vi "Dashboard Main.vi"() -> ()   [LabVIEW 2013]
uses:
  Dropbox/Robot Code old/2014 Target Detection/TargetType.ctl
  <vilib>/event_ctls.llb/eventvkey.ctl
  <vilib>/Rock Robotics/WPI/Dashboard/WPI_DashboardLogging Global.vi
  <vilib>/Utility/config.llb/Write Key (String).vi
  <vilib>/Utility/config.llb/Write Key (I32).vi
  <vilib>/Utility/config.llb/NI_LVConfig.lvlib
panel:
  in  "Camera Type":enum16{"206", "1011", "1013"}(ring)=enum."1013"
  out "Image Message":string="Timeout in Camera Communications"
  in  "Rec Mode":enum32{"Stop", "Record", "Playback"}(radio)
  in  "Dashboard Tab":T1(tab)
  in  "Camera Settings":T2={"Frame Rate"=30, "Compression"=30, "Size"=1} {"Frame Rate" scale=1.0..30.0; "Size" items=["640x480", "320x240", "160x120"]}
  out "MotorSliders R":cluster{"MotorSlide1":dbl, "MotorSlide2":dbl} {"MotorSlide2" scale=-1.0..1.0 scale format="%#_2e"; "MotorSlide1" scale=-1.0..1.0 scale format="%#_2e"}
  out "MotorChart R":cluster{"Numeric":dbl, "Numeric":dbl}(graph)
  out "MotorSliders L":T3 {"MotorSlide4 2" scale=0.0..14.0 scale format="%#_2e"; "MotorSlide2" scale=-1.0..1.0 scale format="%#_2e"; "MotorSlide1" scale=-1.0..1.0 scale format="%#_2e"}
  out "MotorChart L":T4(graph)
  out "JS1 Z":dbl(slide) scale=-1.0..1.0 scale format="%#_2e"
  out "Joystick 1":cluster{"X":dbl, "Y":dbl}[](graph)
  out "JS Buttons 1":T5
  out "JS2 Z":dbl(slide) scale=-1.0..1.0 scale format="%#_2e"
  out "Joystick 2":cluster{"X":dbl, "Y":dbl}[](graph)
  out "JS Buttons 2":T5
  out "Mode":T6(ring)=enum."Auto Disabled"
  out "Camera IP":string
  in  "DB Camera Config":bool
  out "fps":dbl format="%#.1g"
  out "Mbps":dbl format="%#.1g"
  out "Mbps 2":bool
  out "LED 1":bool
  in  "Score Limit":dbl=70.0
  in  "Slider 1":dbl(slide) scale=0.0..100.0
  out "Goal is hot":bool
  out "Distances":T8(array[cluster])
  in  "Color Components":T9={"Hue"={110.0, 142.0}, "Sat"={138.0, 255.0}, "Val"={139.0, 198.0}} {"Val" scale=0.0..255.0; "Sat" scale=0.0..255.0; "Hue" scale=0.0..255.0 scale format="%#_3g"}
  in  "Checkbox 2":bool
  in  "Checkbox 1":bool
  in  "Test Slider":dbl(slide) scale=0.0..100.0 scale format="%#_3g"
  in  "On/Off":bool caption="Solenoid"
  in  "Test Name":u16(ring) items=["Select the test to run...", "Example Test", "-------------------------------", "List of tests is built in robot code.", "Replace with your own automated tests."]
  in  "Test Tree":string(tree)
  in  "Motor":cluster{"Value":dbl, "Enable":bool} {"Value" scale=-1.0..1.0 scale format="%#_3g"}
  out "Progress":T10 {"Test Progress" scale=0.0..100.0}
  in  "Rev/Fwd":cluster{"Forward":bool, "Reverse":bool}
  in  "Test Ring":u16(ring) items=["Auto", "Fixed indoor", "Fixed outdoor 1", "Fixed outdoor 2", "Fixed fluorescent 1", "Fixed fluorescent 2", "Hold current"]
  in  "Listbox":i32(listbox)
  out "Tree":string(tree)
  out "Camera Image":T11(plugin-control)
  in  "Enable":bool
  # "Left"
  # "Front"
  # "Right"
  # "Battery"
  # "Customize by placing controls and indicators here and name to\nmatch Dashboard Variables on robot."
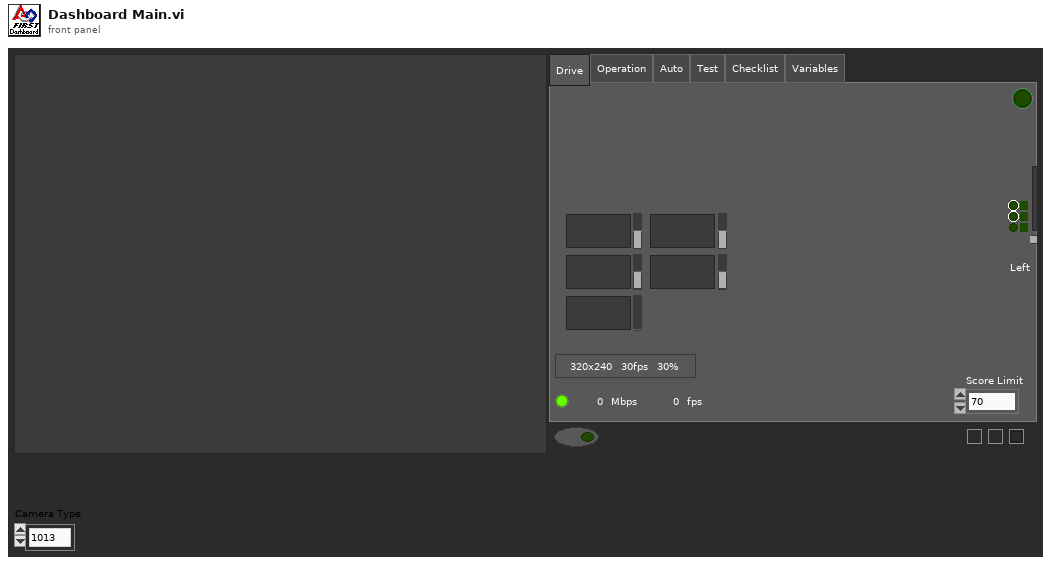
[diagram p1: front panel]
types:
  T1 = enum32{"Drive", "Operation", "Auto", "Test", "Checklist", "Variables"}
  T2 = cluster{"Frame Rate":i32, "Compression":i32, "Size":u16}
  T3 = cluster{"MotorSlide1":dbl, "MotorSlide2":dbl, "MotorSlide4 2":dbl}
  T4 = cluster{"Numeric":dbl, "Numeric":dbl, "Battery":sgl}
  T5 = cluster{bool, bool, bool, bool, bool, bool, bool, bool, bool, bool, bool, bool}
  T6 = enum8{"Tele-Op Disabled", "Tele-Op Enabled", "Auto Disabled", "Auto Enabled", "Test Disabled", "Test Enabled", ""}
  T7 = typedef "TargetType.ctl" = enum16{"Not Hot", "Hot"}
  T8 = cluster{"Distance (ft)":dbl, "Target Center (-1 to 1)":cluster{"X":dbl, "Y":dbl}, "Left":bool, "State":T7}[]
  T9 = cluster{"Hue":cluster{dbl, dbl}, "Sat":cluster{dbl, dbl}, "Val":cluster{dbl, dbl}}
  T10 = cluster{"Test Progress":u8, "Test Progress Text":string}
  T11 = typedef "IMAQ Image.ctl" = refnum<image>
  T12 = typedef "Image Type" = u32
  T13 = cluster{"Digital Inputs":bool[], "Digital Outputs":bool[]}
  T14 = cluster{"Competition mode":bool, "Robot Link":bool, "Autonomous":bool, "Enabled":bool, "E-Stop":bool, "Simulated":bool, "TestMode":bool, "Docked Window":bool}
  T15 = cluster{"Boolean Array[0]":bool, "Boolean Array[1]":bool, "Boolean Array[2]":bool, "Boolean Array[3]":bool, "Boolean Array[4]":bool, "Boolean Array[5]":bool, "Boolean Array[6]":bool, "Boolean Array[7]":bool, "Boolean Array[8]":bool, "Boolean Array[9]":bool, "Boolean Array[10]":bool, "Boolean Array[11]":bool}
  T16 = cluster{"Horizontal":bool, "Aspect Score":dbl, "Rect Score":dbl, cluster{"Left":dbl, "Top":dbl, "Right":dbl, "Bottom":dbl}, "Equiv H":dbl, "Equiv V":dbl}[]
  T17 = cluster{"Scores":cluster{"Total":dbl, "Left":dbl, "Right":dbl, "Ratio":dbl, "Vertical":dbl, "index":i32, "State":T7}, "Verticals":cluster{"Horizontal?":bool, "Aspect Score":dbl, "Rect Score":dbl, cluster{"Left":dbl, "Top":dbl, "Right":dbl, "Bottom":dbl}, "Equiv H":dbl, "Equiv V":dbl}, "Horizontals":cluster{"Horizontal?":bool, "Aspect Score":dbl, "Rect Score":dbl, cluster{"Left":dbl, "Top":dbl, "Right":dbl, "Bottom":dbl}, "Equiv H":dbl, "Equiv V":dbl}, "Validated":bool}[]
  T18 = cluster{"Scores":cluster{"Total":dbl, "Left":dbl, "Right":dbl, "Ratio":dbl, "Vertical":dbl, "index":i32, "State":T7}, "Verticals":cluster{"Horizontal?":bool, "Aspect Score":dbl, "Rect Score":dbl, cluster{"Left":dbl, "Top":dbl, "Right":dbl, "Bottom":dbl}, "Equiv H":dbl, "Equiv V":dbl}, "Horizontals":cluster{"Horizontal?":bool, "Aspect Score":dbl, "Rect Score":dbl, cluster{"Left":dbl, "Top":dbl, "Right":dbl, "Bottom":dbl}, "Equiv H":dbl, "Equiv V":dbl}, "Distance (ft)":dbl, "Target Center (-1 to 1)":cluster{"X":dbl, "Y":dbl}}[]
  T19 = cluster{"Target Info[0]":cluster{"Scores":cluster{"Total":dbl, "Left":dbl, "Right":dbl, "Ratio":dbl, "Vertical":dbl, "index":i32, "State":T7}, "Verticals":cluster{"Horizontal?":bool, "Aspect Score":dbl, "Rect Score":dbl, cluster{"Left":dbl, "Top":dbl, "Right":dbl, "Bottom":dbl}, "Equiv H":dbl, "Equiv V":dbl}, "Horizontals":cluster{"Horizontal?":bool, "Aspect Score":dbl, "Rect Score":dbl, cluster{"Left":dbl, "Top":dbl, "Right":dbl, "Bottom":dbl}, "Equiv H":dbl, "Equiv V":dbl}, "Distance (ft)":dbl, "Target Center (-1 to 1)":cluster{"X":dbl, "Y":dbl}}, "Target Info[1]":cluster{"Scores":cluster{"Total":dbl, "Left":dbl, "Right":dbl, "Ratio":dbl, "Vertical":dbl, "index":i32, "State":T7}, "Verticals":cluster{"Horizontal?":bool, "Aspect Score":dbl, "Rect Score":dbl, cluster{"Left":dbl, "Top":dbl, "Right":dbl, "Bottom":dbl}, "Equiv H":dbl, "Equiv V":dbl}, "Horizontals":cluster{"Horizontal?":bool, "Aspect Score":dbl, "Rect Score":dbl, cluster{"Left":dbl, "Top":dbl, "Right":dbl, "Bottom":dbl}, "Equiv H":dbl, "Equiv V":dbl}, "Distance (ft)":dbl, "Target Center (-1 to 1)":cluster{"X":dbl, "Y":dbl}}, "Target Info[2]":cluster{"Scores":cluster{"Total":dbl, "Left":dbl, "Right":dbl, "Ratio":dbl, "Vertical":dbl, "index":i32, "State":T7}, "Verticals":cluster{"Horizontal?":bool, "Aspect Score":dbl, "Rect Score":dbl, cluster{"Left":dbl, "Top":dbl, "Right":dbl, "Bottom":dbl}, "Equiv H":dbl, "Equiv V":dbl}, "Horizontals":cluster{"Horizontal?":bool, "Aspect Score":dbl, "Rect Score":dbl, cluster{"Left":dbl, "Top":dbl, "Right":dbl, "Bottom":dbl}, "Equiv H":dbl, "Equiv V":dbl}, "Distance (ft)":dbl, "Target Center (-1 to 1)":cluster{"X":dbl, "Y":dbl}}, "Target Info[3]":cluster{"Scores":cluster{"Total":dbl, "Left":dbl, "Right":dbl, "Ratio":dbl, "Vertical":dbl, "index":i32, "State":T7}, "Verticals":cluster{"Horizontal?":bool, "Aspect Score":dbl, "Rect Score":dbl, cluster{"Left":dbl, "Top":dbl, "Right":dbl, "Bottom":dbl}, "Equiv H":dbl, "Equiv V":dbl}, "Horizontals":cluster{"Horizontal?":bool, "Aspect Score":dbl, "Rect Score":dbl, cluster{"Left":dbl, "Top":dbl, "Right":dbl, "Bottom":dbl}, "Equiv H":dbl, "Equiv V":dbl}, "Distance (ft)":dbl, "Target Center (-1 to 1)":cluster{"X":dbl, "Y":dbl}}, "Target Info[4]":cluster{"Scores":cluster{"Total":dbl, "Left":dbl, "Right":dbl, "Ratio":dbl, "Vertical":dbl, "index":i32, "State":T7}, "Verticals":cluster{"Horizontal?":bool, "Aspect Score":dbl, "Rect Score":dbl, cluster{"Left":dbl, "Top":dbl, "Right":dbl, "Bottom":dbl}, "Equiv H":dbl, "Equiv V":dbl}, "Horizontals":cluster{"Horizontal?":bool, "Aspect Score":dbl, "Rect Score":dbl, cluster{"Left":dbl, "Top":dbl, "Right":dbl, "Bottom":dbl}, "Equiv H":dbl, "Equiv V":dbl}, "Distance (ft)":dbl, "Target Center (-1 to 1)":cluster{"X":dbl, "Y":dbl}}, "Target Info[5]":cluster{"Scores":cluster{"Total":dbl, "Left":dbl, "Right":dbl, "Ratio":dbl, "Vertical":dbl, "index":i32, "State":T7}, "Verticals":cluster{"Horizontal?":bool, "Aspect Score":dbl, "Rect Score":dbl, cluster{"Left":dbl, "Top":dbl, "Right":dbl, "Bottom":dbl}, "Equiv H":dbl, "Equiv V":dbl}, "Horizontals":cluster{"Horizontal?":bool, "Aspect Score":dbl, "Rect Score":dbl, cluster{"Left":dbl, "Top":dbl, "Right":dbl, "Bottom":dbl}, "Equiv H":dbl, "Equiv V":dbl}, "Distance (ft)":dbl, "Target Center (-1 to 1)":cluster{"X":dbl, "Y":dbl}}, "Target Info[6]":cluster{"Scores":cluster{"Total":dbl, "Left":dbl, "Right":dbl, "Ratio":dbl, "Vertical":dbl, "index":i32, "State":T7}, "Verticals":cluster{"Horizontal?":bool, "Aspect Score":dbl, "Rect Score":dbl, cluster{"Left":dbl, "Top":dbl, "Right":dbl, "Bottom":dbl}, "Equiv H":dbl, "Equiv V":dbl}, "Horizontals":cluster{"Horizontal?":bool, "Aspect Score":dbl, "Rect Score":dbl, cluster{"Left":dbl, "Top":dbl, "Right":dbl, "Bottom":dbl}, "Equiv H":dbl, "Equiv V":dbl}, "Distance (ft)":dbl, "Target Center (-1 to 1)":cluster{"X":dbl, "Y":dbl}}, "Target Info[7]":cluster{"Scores":cluster{"Total":dbl, "Left":dbl, "Right":dbl, "Ratio":dbl, "Vertical":dbl, "index":i32, "State":T7}, "Verticals":cluster{"Horizontal?":bool, "Aspect Score":dbl, "Rect Score":dbl, cluster{"Left":dbl, "Top":dbl, "Right":dbl, "Bottom":dbl}, "Equiv H":dbl, "Equiv V":dbl}, "Horizontals":cluster{"Horizontal?":bool, "Aspect Score":dbl, "Rect Score":dbl, cluster{"Left":dbl, "Top":dbl, "Right":dbl, "Bottom":dbl}, "Equiv H":dbl, "Equiv V":dbl}, "Distance (ft)":dbl, "Target Center (-1 to 1)":cluster{"X":dbl, "Y":dbl}}, "Target Info[8]":cluster{"Scores":cluster{"Total":dbl, "Left":dbl, "Right":dbl, "Ratio":dbl, "Vertical":dbl, "index":i32, "State":T7}, "Verticals":cluster{"Horizontal?":bool, "Aspect Score":dbl, "Rect Score":dbl, cluster{"Left":dbl, "Top":dbl, "Right":dbl, "Bottom":dbl}, "Equiv H":dbl, "Equiv V":dbl}, "Horizontals":cluster{"Horizontal?":bool, "Aspect Score":dbl, "Rect Score":dbl, cluster{"Left":dbl, "Top":dbl, "Right":dbl, "Bottom":dbl}, "Equiv H":dbl, "Equiv V":dbl}, "Distance (ft)":dbl, "Target Center (-1 to 1)":cluster{"X":dbl, "Y":dbl}}}
  T20 = cluster{cluster{dbl, dbl}, cluster{dbl, dbl}, cluster{dbl, dbl}}
  T21 = typedef "NI_LVConfig.lvlib/Config Data RefNum.ctl" = refnum<k1>
  T22 = typedef "eventvkey.ctl" = enum16{"ASCII", "Enter", "Return", "Shift", "Ctrl", "Alt", "Cmd", "Opt", "Caps", "NumLock", "Clear", "Break", "Up", "Down", "Left", "Right", "Insert", "Delete", "Home", "End", "PageUp", "PageDown", "Escape", "Help", "Pause", "ScrollLock", "F1", "F2", "F3", "F4", "F5", "F6", "F7", "F8", "F9", "F10", "F11", "F12", "F13", "F14", "F15", "F16", "F17", "F18", "F19", "F20", "F21", "F22", "F23", "F24", "Play", "VolumeUp", "VolumeDown", "Mute", "Two Byte Char"}
  T23 = cluster{"Image Size":bool, "Image Type":bool, "Pixel Value":bool, "ROI Information":bool, "Zoom Factor":bool}
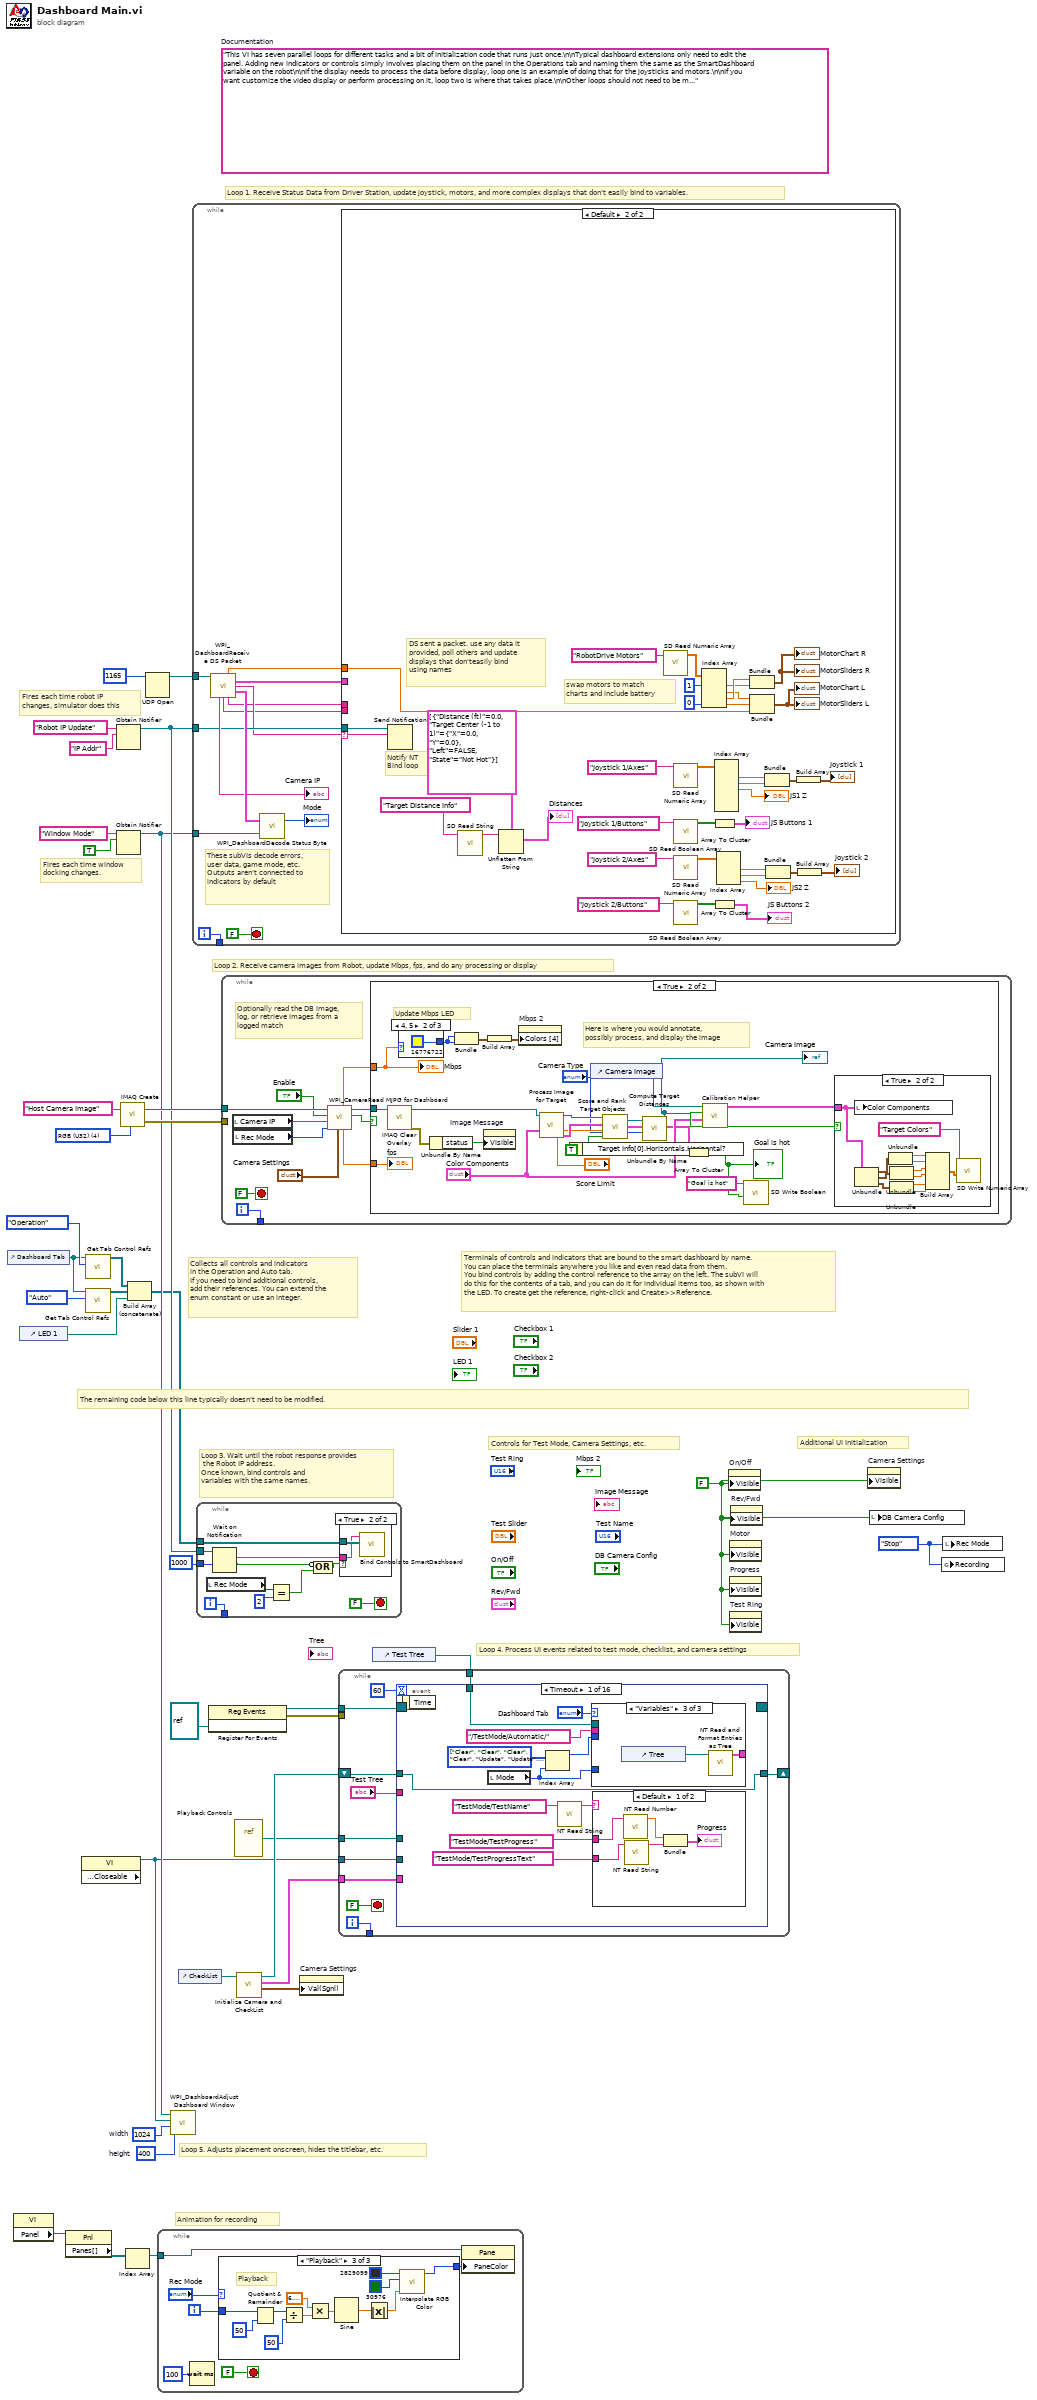
[diagram p0: block diagram]
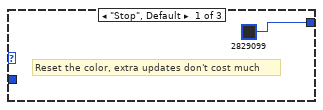
[diagram p2: hidden frame]
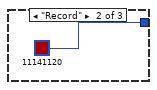
[diagram p3: hidden frame]
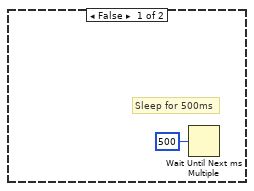
[diagram p5: hidden frame]
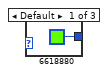
[diagram p7: hidden frame]
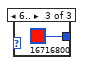
[diagram p8: hidden frame]
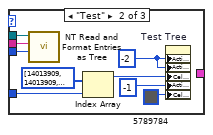
[diagram p10: hidden frame]
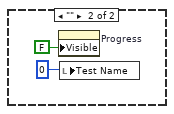
[diagram p11: hidden frame]
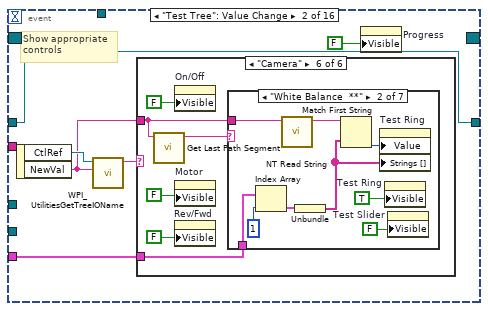
[diagram p12: hidden frame]
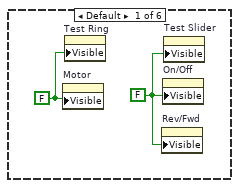
[diagram p13: hidden frame]
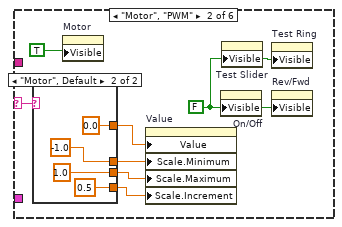
[diagram p14: hidden frame]
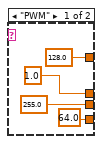
[diagram p15: hidden frame]
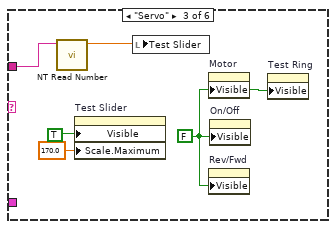
[diagram p16: hidden frame]
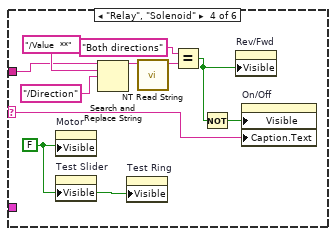
[diagram p17: hidden frame]
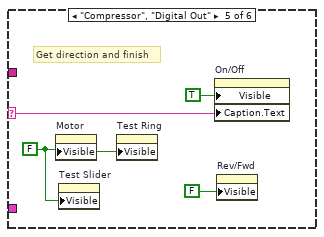
[diagram p18: hidden frame]
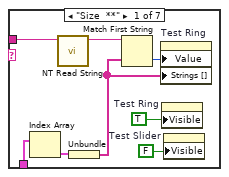
[diagram p19: hidden frame]
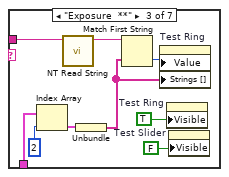
[diagram p20: hidden frame]
diagram:
  w8 = enum32{"Stop", "Record", "Playback"}."Stop" ("Rec Mode")
  w11 = 400  # height
  w12 = 1024  # width
  w25 = FALSE ("Visible")
  (unwired) "This VI has seven parallel loops for different tasks and a bit of initialization code that runs just once.\n\nTypical dashboard extensions only need to edit the panel. Adding new indicators or controls simply involves placing them on the panel in the Operations tab and naming them the same as the SmartDashboard variable on the robot\n\nIf the display needs to process the data before display, loop one is an example of doing that for the joysticks and motors.\n\nIf you want customize the video display or perform processing on it, loop two is where that takes place.\n\nOther loops should not need to be modified. They are pretty standard, and document the task they perform."  # Documentation
  w35 = T12 4 items=["Grayscale (U8)", "Grayscale (I16)", "Grayscale (SGL)", "Complex (CSG)", "RGB (U32)", "HSL (U32)", "RGB (U64)"] ("Image Type")
  # "Controls for Test Mode, Camera Settings, etc."
  # "Additional UI Initialization"
  # "Animation for recording"
  # "Fires each time robot IP\nchanges, simulator does this"
  # "Fires each time window\ndocking changes."
  # "Collects all controls and indicators\nin the Operation and Auto tab.\nIf you need to bind additional controls,\nadd their references. You can extend the\nenum constant or use an integer."
  # "The remaining code below this line typically doesn't need to be modified."
  # "Loop 4. Process UI events related to test mode, checklist, and camera settings"
  # "Terminals of controls and indicators that are bound to the smart dashboard by name.\nYou can place the terminals anywhere you like and even read data from them.\nYou bind controls by adding the control reference to the array on the left. The subVI will\ndo this for the contents of a tab, and you can do it for individual items too, as shown with\nthe LED. To create get the reference, right-click and Create>>Reference."
  # "Loop 3. Wait until the robot response provides\n the Robot IP address.\nOnce known, bind controls and\nvariables with the same names."
  # "Loop 5. Adjusts placement onscreen, hides the titlebar, etc."
  # "Loop 1. Receive Status Data from Driver Station, update joystick, motors, and more complex displays that don't easily bind to variables."
  # "Loop 2. Receive camera images from Robot, update Mbps, fps, and do any processing or display"
  n1 = control-ref of="Dashboard Tab"() -> (w6:refnum<vi>)
  n2 = property class="VI"() -> ("Panel"=w19:refnum<vi>)  [unwired: 2 in, 2 out]
  n3 = control-ref of="LED 1"() -> (w1:refnum<vi>)
  n4 = property class="Pnl"(reference=w19) -> ("Panes[]"=w20:refnum<vi>[])  [unwired: 1 in, 2 out]
  n5 = property class="VI" props=["Front Panel.Closeable"]() -> (reference out=w7:refnum<vi>)  [unwired: 2 in, 2 out]
  n6 = call <vilib>:"Get Tab Control Refs.vi"("Page Index"=T1."Operation" ("Dashboard Tab"), "TabControl in"=w6) -> ("ControlsOnPage"=w4:refnum<vi>[])  [unwired: 9 in]
  n7 = call <vilib>:"Get Tab Control Refs.vi"("Page Index"=T1."Auto" ("Dashboard Tab"), "TabControl in"=w6) -> ("ControlsOnPage"=w5:refnum<vi>[])  [unwired: 9 in]
  n8 = Obtain Notifier(name (unnamed)="Robot IP Update", notification data type="IP Addr" ("name (unnamed)")) -> (notifier out=w29:refnum<notifier>)  [unwired: 2 in, 2 out]
  n9 = Obtain Notifier(name (unnamed)="Window Mode", notification data type=TRUE) -> (notifier out=w10:refnum<notifier>)  [unwired: 2 in, 2 out]
  n10 = call "IMAQ Create"("Image Name"="Host Camera Image", "Image Type"=w35) -> ("New Image"=w33:T11, "error out"=w32:errorcluster)  [unwired: 2 in, 1 out]
  n11 = Index Array(array=w20) -> (element=w18:refnum<vi>)  [unwired: 1 in]
  n12 = Build Array (concatenate)(w4, w5, w1) -> (w3:refnum<vi>[])
  n13 = UDP Open(11:u16 1165 ("port")) -> (port=w36:refnum<k16>)  [unwired: 2 in, 4 out]
  n14 = while {
    tunnel: w18 -> [w39]
    i -> [w42]
    stop <- FALSE stop-if-true
    n15 = Wait (ms)(milliseconds to wait=u32 100) -> ()  [unwired: 1 out]
    n16 = case shown="\"Playback\"" "Rec Mode" {
      tunnel: w42 -> [_ _ w57]
      tunnel: [u32 2829099 ("Base Color") u32 11141120 ("Target Color") w46] -> w38
      frame "Stop", Default {
        # "Reset the color, extra updates don't cost much"
      }
      frame "Record" {
      }
      frame "Playback" {
        # "Playback"
        n17 = Quotient & Remainder(x=w57, y=u32 50 ("milliseconds to wait")) -> (x-y*floor(x/y)=w53:u32)  [unwired: 1 out]
        n18 = Divide(x=w53, y=u32 50 ("milliseconds to wait")) -> (x/y=w50:dbl)
        n19 = Multiply(x=6.283185307179586, y=w50) -> (x*y=w55:dbl)
        n20 = Sine(x=w55) -> (sin(x)=w54:dbl)
        n21 = Absolute Value(x=w54) -> (abs(x)=w47:dbl)
        n22 = call "Interpolate RGB Color.vi"("Proportion"=w47, "Target Color"=u32 30976, "Base Color"=u32 2829099) -> ("Result Color"=w46:u32)  [unwired: 8 in]
      }
    }
    n23 = property class="Pane"(reference=w39, "PaneColor"=w38) -> ()  [unwired: 1 in, 2 out]
  }
  n24 = call <vilib>:"WPI_DashboardAdjust Dashboard Window.vi"("height"=w11, "width"=w12, "reference in"=w7, "Notifier in"=w10) -> ()  [unwired: 8 in]
  n25 = control-ref of="CheckList"() -> (w9:refnum<vi>)
  n26 = while {
    tunnel: w36 -> [w68]
    tunnel: w29 -> [w63]
    tunnel: w10 -> [w67]
    tunnel: [w64] -> _
    i -> [w64]
    stop <- FALSE stop-if-true
    # "These subVIs decode errors, user data, game mode, etc.\nOutputs aren't connected to indicators by default"
    n27 = call <vilib>:"WPI_DashboardReceive DS Packet.vi"("Recv Socket"=w68) -> ("Battery"=w58:sgl, "Driver Station"=w59:T13, "Robot IP Address"=w62:string, "Status"=w69:T14, "Camera IP Address"=→"Camera IP":string, "Low Priority User Data"=w61:string, "High Priority User Data"=w60:string)  [unwired: 1 in, 7 out]
    n28 = call <vilib>:"WPI_DashboardDecode Status Byte.vi"("Window Mode Notifier"=w67, "Status"=w69) -> ("Mode"=→"Mode":T6)  [unwired: 1 out]
    n29 = case shown="Default" w62 {
      selector: w62 -> [_ w85]
      tunnel: w63 -> [_ w86]
      tunnel: w61 -> [_ _]
      tunnel: w60 -> [_ _]
      tunnel: w59 -> [_ _]
      tunnel: w58 -> [_ w84]
      frame "0.0.0.0" {
        # "DS not sending packets, or no robot exists yet.\nDon't poll the variables"
      }
      frame Default {
        # "Notify NT\nBind loop"
        # "DS sent a packet. use any data it\nprovided, poll others and update\ndisplays that don'teasily bind\nusing names"
        # "swap motors to match\ncharts and include battery"
        n30 = Send Notification(notification=w85, notifier=w86) -> ()  [unwired: 1 in, 2 out]
        n31 = call <vilib>:"SD Read String.vi"("Name"="Target Distance Info") -> ("String"=w74:string)  [unwired: 8 in, 2 out]
        n32 = Unflatten From String(type=T8 [{"Distance (ft)"=0.0, "Target Center (-1 to 1)"={"X"=0.0, "Y"=0.0}, "Left"=FALSE, "State"=enum."Not Hot"}] ("Distances"), binary string=w74) -> (value=→"Distances":T8)  [unwired: 3 in, 2 out]
        n33 = call <vilib>:"SD Read Numeric Array.vi"("Name"="RobotDrive Motors") -> ("Numeric Array"=w83:dbl[])  [unwired: 8 in, 2 out]
        n34 = call <vilib>:"SD Read Numeric Array.vi"("Name"="Joystick 1/Axes") -> ("Numeric Array"=w102:dbl[])  [unwired: 8 in, 2 out]
        n35 = call <vilib>:"SD Read Boolean Array.vi"("Name"="Joystick 1/Buttons") -> ("Boolean Array"=w104:bool[])  [unwired: 8 in, 2 out]
        n36 = call <vilib>:"SD Read Numeric Array.vi"("Name"="Joystick 2/Axes") -> ("Numeric Array"=w96:dbl[])  [unwired: 8 in, 2 out]
        n37 = call <vilib>:"SD Read Boolean Array.vi"("Name"="Joystick 2/Buttons") -> ("Boolean Array"=w95:bool[])  [unwired: 8 in, 2 out]
        n38 = Index Array(array=w83, index #1=1, index #4=0) -> (element #1=w79:dbl, element #2=w78:dbl, element #3=w80:dbl, element #4=w75:dbl)  [unwired: 2 in]
        n39 = Array To Cluster(array=w104) -> (cluster=→"JS Buttons 1":T15)
        n40 = Array To Cluster(array=w95) -> (cluster=→"JS Buttons 2":T15)
        n41 = Index Array(array=w102) -> (element #1=w99:dbl, element #2=w100:dbl, element #3=→"JS1 Z":dbl)  [unwired: 6 in, 3 out]
        n42 = Index Array(array=w96) -> (element #1=w91:dbl, element #2=w90:dbl, element #3=→"JS2 Z":dbl)  [unwired: 3 in]
        n43 = Bundle("Numeric"=w80, "Numeric"=w79) -> (→"MotorChart R" →"MotorSliders R":cluster{"Numeric":dbl, "Numeric":dbl})  [unwired: 1 in]
        n44 = Bundle("Numeric"=w78, "Numeric"=w75, "Battery"=w84) -> (→"MotorChart L" →"MotorSliders L":T4)  [unwired: 1 in]
        n45 = Bundle("Numeric"=w99, "Numeric"=w100) -> (w98:cluster{"Numeric":dbl, "Numeric":dbl})  [unwired: 1 in]
        n46 = Bundle("Numeric"=w91, "Numeric"=w90) -> (w92:cluster{"Numeric":dbl, "Numeric":dbl})  [unwired: 1 in]
        n47 = Build Array(w98) -> (→"Joystick 1":cluster{"Numeric":dbl, "Numeric":dbl}[])
        n48 = Build Array(w92) -> (→"Joystick 2":cluster{"Numeric":dbl, "Numeric":dbl}[])
      }
    }
  }
  n49 = while {
    tunnel: w3 -> [w118]
    tunnel: w29 -> [w116]
    tunnel: [w114] -> _
    tunnel: u32 1000 ("milliseconds to wait") -> [w113]
    i -> [w114]
    stop <- FALSE stop-if-true
    n50 = local read "Rec Mode"() -> (w109:enum32{"Stop", "Record", "Playback"})
    n51 = Wait on Notification(notifier=w116, timeout in ms (-1)=w113) -> (notification=w115:string, timed out?=w111:bool)  [unwired: 2 in, 2 out]
    n52 = Equal?(x=w109, y=u16 2 ("Rec Mode")) -> (x = y?=w110:bool)
    n53 = Compound Arithmetic op=OR(invert w111, w110) -> (w112:bool)
    n54 = case shown="True" w112 {
      tunnel: w118 -> [_ w120]
      tunnel: w115 -> [_ w119]
      frame False {
      }
      frame True {
        n55 = call <vilib>:"Bind Controls to SmartDashboard.vi"("Bound Control Refs"=w120, "Server IP Address"=w119) -> ()  [unwired: 10 in]
      }
    }
  }
  n56 = register-events(refnum<vi> refnum) -> (reference out=w16:refnum<event-registration>, error out=w15:errorcluster)  [unwired: 2 in]
  n57 = while {
    tunnel: w33 -> [w129]
    tunnel: w32 -> [_]
    tunnel: [w130] -> _
    i -> [w130]
    stop <- FALSE stop-if-true
    # "Optionally read the DB image,\nlog, or retrieve images from a\nlogged match"
    n58 = local read "Camera IP"() -> (w122:string)
    n59 = local read "Rec Mode"() -> (w121:enum32{"Stop", "Record", "Playback"})
    n60 = call <vilib>:"WPI_CameraRead MJPG for Dashboard.vi"("Camera Settings"="Camera Settings", "Rec Mode"=w121, "Camera IP"=w122, "Enable"="Enable", "Refnum in"=w129) -> ("Active"=w126:bool, "Refnum out"=w128:T11, "FPS"=w125:dbl, "Bandwidth (Mbps)"=w124:dbl)  [unwired: 3 in]
    n61 = case shown="True" w126 {
      tunnel: w128 -> [_ w152]
      tunnel: w124 -> [_ w151]
      tunnel: w125 -> [_ w150]
      frame False {
        # "Sleep for 500ms"
        n62 = Wait Until Next ms Multiple(millisecond multiple=u32 500) -> ()  [unwired: 1 out]
      }
      frame True {
        # "Here is where you would annotate,\npossibly process, and display the image"
        # "Update Mbps LED"
        n63 = call "IMAQ Clear Overlay"("Image"=w152) -> ("error out"=w156:errorcluster, "Image Out"=w145:T11)  [unwired: 2 in, 7 out]
        n64 = case shown="4, 5" w151 {
          tunnel: [u32 6618880 ("Color Box") u32 16776722 ("Color Box") u32 16716800 ("Color Box")] -> w153
          frame Default {
          }
          frame 4, 5 {
          }
          frame 6.. {
          }
        }
        n65 = Unbundle By Name(w156) -> ("status"=w157:bool)
        n66 = Bundle("Color Box"=w153, "Color Box"=w153) -> (w155:cluster{"Color Box":u32, "Color Box":u32})  [unwired: 1 out]
        n67 = property on="Image Message" class="Str"("Visible"=w157) -> ()  [unwired: 2 in, 2 out]
        n68 = Build Array(w155) -> (w154:cluster{"Color Box":u32, "Color Box":u32}[])
        n69 = property on="Mbps 2" class="Bool (strict)"("Colors [4]"=w154) -> ()  [unwired: 2 in, 2 out]
        n70 = call "Process Image for Target.vi"("Src Image"=w145, "Color Components"="Color Components") -> ("Src Image Out"=w144:T11, "Particles"=w143:T16)  [unwired: 11 in, 1 out]
        n71 = control-ref of="Camera Image"() -> (w149:refnum<vi>)
        n72 = call "Score and Rank Target Objects.vi"("Annotate"=TRUE, "Score Limit"="Score Limit", "Particles"=w143, "Image in"=w144) -> ("Target Info"=w142:T17, "Annotated Image"=w141:T11)  [unwired: 6 in]
        n73 = call "Compute Target Distances.vi"("Camera Type"="Camera Type", "Target Info"=w142, "Image in"=w141) -> ("Target Info"=w136:T18, "Image out"=w140:T11)  [unwired: 6 in, 1 out]
        "Camera Image" <- w140
        n74 = Array To Cluster(array=w136) -> (cluster=w135:T19)
        n75 = Unbundle By Name(w135) -> ("Target Info[0].Horizontals.Horizontal?"=w134:bool)
        "Goal is hot" <- w134
        n76 = call "Calibration Helper.vi"("Color Components"="Color Components", "Image"=w140, "Image Ctl Refnum"=w149) -> ("Changed"=w147:bool, "output color"=w148:T20)  [unwired: 7 in]
        n77 = call <vilib>:"SD Write Boolean.vi"("Boolean"=w134, "Name"="Goal is hot") -> ()  [unwired: 8 in, 2 out]
        n78 = case shown="True" w147 {
          tunnel: w148 -> [_ w169]
          frame False {
          }
          frame True {
            n79 = local write "Color Components"(w169) -> ()
            n80 = Unbundle(w169) -> (w168:cluster{dbl, dbl}, w167:cluster{dbl, dbl}, w166:cluster{dbl, dbl})
            n81 = Unbundle(w168) -> (w165:dbl, w164:dbl)
            n82 = Unbundle(w167) -> (w163:dbl, w162:dbl)
            n83 = Unbundle(w166) -> (w161:dbl, w160:dbl)
            n84 = Build Array(w165, w164, w163, w162, w161, w160) -> (w159:dbl[])
            n85 = call <vilib>:"SD Write Numeric Array.vi"("Numeric Array"=w159, "Name"="Target Colors") -> ()  [unwired: 8 in, 2 out]
          }
        }
        "Mbps" <- w151
        "fps" <- w150
      }
    }
  }
  n86 = vi-ref "Playback Controls.vi"() -> (w17:refnum<vi>)
  n87 = call "Initialize Camera and CheckList.vi"("ListBox in"=w9) -> ("Cluster"=w23:cluster{"value":i32, "value":i32, "index":i32}, "Array"=w24:cluster{string[]}[], "File Refnum"=w22:T21)  [unwired: 8 in]
  n88 = property on="Camera Settings" class="Clust (strict)"("Val(Sgnl)"=w23) -> ()  [unwired: 2 in, 2 out]
  n89 = control-ref of="Test Tree"() -> (w21:refnum<vi>)
  n90 = while {
    tunnel: w24 -> [w180]
    shift-right: [w179] -> _
    shift-left: w22 -> [w178]
    tunnel: [w177] -> _
    tunnel: w21 -> [w176]
    tunnel: w17 -> [w175]
    tunnel: w16 -> [w174]
    tunnel: w15 -> [_]
    tunnel: w7 -> [w173]
    i -> [w177]
    stop <- FALSE stop-if-true
    n91 = event shown="[0] Timeout" {
      selector: w174 -> [_ _ _ _ _ _ _ _ _ _ _ _ _ _ _ _]
      dyn-events: [_ _ _ _ _ _ _ _ _ _ _ _ _ w418 _ _] -> _
      timeout: u32 60 ("milliseconds to wait") -> [_ _ _ _ _ _ _ _ _ _ _ _ _ _ _ _]
      tunnel: w176 -> [w190 _ _ _ _ _ _ _ _ _ _ _ _ _ _ _]
      tunnel: "Test Tree" -> [_ _ _ _ _ _ _ _ w387 w395 w397 w401 w409 _ _ _]
      tunnel: w180 -> [_ w214 _ _ _ _ w351 w381 _ _ _ _ _ _ _ _]
      tunnel: [w184 w213 w312 w317 w325 w337 w350 w374 w386 w393 w396 w400 w408 w420 w434 w435] -> w179
      tunnel: w178 -> [w184 w213 w312 w317 w325 w337 w349 w374 w386 w393 w396 w400 w408 w420 w434 w435]
      tunnel: w175 -> [_ _ _ _ _ _ _ _ _ _ _ _ _ w421 _ w438]
      tunnel: w173 -> [_ _ _ _ _ _ _ _ _ _ _ _ _ w416 _ _]
      event Timeout {
        w189 = enum16{"Update", "Clear"}[] [enum."Clear", enum."Clear", enum."Clear", enum."Clear", enum."Update", enum."Update", enum."Clear"] items=["Update", "Clear"]
        n92 = event-data() -> ()  [unwired: 1 in, 1 out]
        n93 = local read "Mode"() -> (w187:T6)
        n94 = Index Array(array=w189, index=w187) -> (element=w188:enum16{"Update", "Clear"})
        n95 = call <vilib>:"NT Read String.vi"("Name"="TestMode/TestName") -> ("String"=w193:string)  [unwired: 9 in, 1 out]
        n96 = case shown="\"Variables\"" "Dashboard Tab" {
          tunnel: w190 -> [_ w203 _]
          tunnel: "/TestMode/Automatic/" ("Name Pattern") -> [_ w202 _]
          tunnel: w188 -> [_ w201 _]
          tunnel: w187 -> [_ w199 _]
          tunnel: [_ _ w205] -> _
          frame "Operation", Default {
          }
          frame "Test" {
            w198 = -2 ("Active Item:Row Number")
            n97 = call <vilib>:"NT Read and Format Entries as Tree.vi"("Operation"=w201, "Name Pattern"=w202, "Tree Refnum"=w203) -> ()  [unwired: 7 in, 2 out]
            n98 = Index Array(array=u32[] [14013909, 14013909, 14013909, 14013909, 14013909, 16777215, 14013909], index=w199) -> (element=w197:u32)
            n99 = property on="Test Tree" class="Tree (strict)"("Active Item Row Number"=w198, "ActiveColNum"=w198, "CellBG"=w197, "Active Item Row Number"=-1 ("Active Item:Row Number"), "CellBG"=u32 5789784 ("Color Box")) -> ()  [unwired: 2 in, 2 out]
          }
          frame "Variables" {
            n100 = control-ref of="Tree"() -> (w204:refnum<vi>)
            n101 = call <vilib>:"NT Read and Format Entries as Tree.vi"("Tree Refnum"=w204) -> ("Formatted Strings"=w205:cluster{"Name":string, "Value":string}[])  [unwired: 9 in, 1 out]
          }
        }
        n102 = case shown="Default" w193 {
          tunnel: "TestMode/TestProgress" ("Name") -> [w207 _]
          tunnel: "TestMode/TestProgressText" ("Name") -> [w206 _]
          frame Default {
            n103 = call <vilib>:"NT Read Number.vi"("Name"=w207) -> ("Numeric"=w208:dbl)  [unwired: 9 in, 1 out]
            n104 = call <vilib>:"NT Read String.vi"("Name"=w206) -> ("String"=w209:string)  [unwired: 9 in, 1 out]
            n105 = Bundle("Numeric"=w208, "String"=w209) -> (→"Progress":cluster{"Numeric":dbl, "String":string})  [unwired: 1 in]
          }
          frame "" {
            n106 = property on="Progress" class="Clust (strict)"("Visible"=FALSE) -> ()  [unwired: 2 in, 2 out]
            n107 = local write "Test Name"(u16 0) -> ()
          }
        }
      }
      event "Test Tree": Value Change {
        # "Show appropriate\ncontrols"
        n108 = event-data() -> ("CtlRef"=w217:refnum<vi>, "NewVal"=w215:string)  [unwired: 1 in]
        n109 = call <vilib>:"WPI_UtilitiesGetTreeIOName.vi"("NewVal"=w215, "TreeControl in"=w217) -> ("I/O Name"=w218:string)  [unwired: 9 in]
        n110 = case shown="\"Camera\"" w218 {
          selector: w218 -> [_ w225 _ w243 w252 _]
          tunnel: w215 -> [_ _ w240 w242 _ w259]
          tunnel: w214 -> [_ _ _ _ _ w258]
          frame Default {
            w220 = FALSE ("Visible")
            w219 = FALSE ("Visible")
            n111 = property on="Motor" class="Clust (strict)"("Visible"=w219) -> ()  [unwired: 2 in, 2 out]
            n112 = property on="Test Ring" class="Ring (strict)"("Visible"=w219) -> ()  [unwired: 2 in, 2 out]
            n113 = property on="Rev/Fwd" class="Clust (strict)"("Visible"=w220) -> ()  [unwired: 2 in, 2 out]
            n114 = property on="On/Off" class="Bool (strict)"("Visible"=w220) -> ()  [unwired: 2 in, 2 out]
            n115 = property on="Test Slider" class="Slide (strict)"("Visible"=w220) -> ()  [unwired: 2 in, 2 out]
          }
          frame "Motor", "PWM" {
            w226 = FALSE ("Visible")
            n116 = case shown="\"Motor\", Default" w225 {
              tunnel: [1.0 ("Value") -1.0 ("Value")] -> w224
              tunnel: [255.0 ("Value") 1.0 ("Value")] -> w223
              tunnel: [128.0 ("Value") 0.0 ("Value")] -> w222
              tunnel: [64.0 ("Value") 0.5 ("Value")] -> w221
              frame "PWM" {
              }
              frame "Motor", Default {
              }
            }
            n117 = property on="Motor" class="Clust (strict)"("Visible"=TRUE) -> ()  [unwired: 2 in, 2 out]
            n118 = property on="Value" class="Slide (strict)"("Value"=w222, "Scale.Minimum"=w224, "Scale.Maximum"=w223, "Scale.Increment"=w221) -> ()  [unwired: 2 in, 2 out]
            n119 = property on="On/Off" class="Bool (strict)"("Visible"=w226) -> ()  [unwired: 2 in, 2 out]
            n120 = property on="Test Slider" class="Slide (strict)"("Visible"=w226) -> ()  [unwired: 2 in, 2 out]
            n121 = property on="Test Ring" class="Ring (strict)"("Visible"=w226) -> ()  [unwired: 2 in, 2 out]
            n122 = property on="Rev/Fwd" class="Clust (strict)"("Visible"=w226) -> ()  [unwired: 2 in, 2 out]
          }
          frame "Servo" {
            w238 = FALSE ("Visible")
            n123 = call <vilib>:"NT Read Number.vi"("Name"=w240) -> ("Numeric"=w239:dbl)  [unwired: 9 in, 1 out]
            n124 = property on="Test Slider" class="Slide (strict)"("Visible"=TRUE, "Scale.Maximum"=170.0 ("Scale.Range:Maximum")) -> ()  [unwired: 2 in, 2 out]
            n125 = local write "Test Slider"(w239) -> ()
            n126 = property on="Motor" class="Clust (strict)"("Visible"=w238) -> ()  [unwired: 2 in, 2 out]
            n127 = property on="Rev/Fwd" class="Clust (strict)"("Visible"=w238) -> ()  [unwired: 2 in, 2 out]
            n128 = property on="On/Off" class="Bool (strict)"("Visible"=w238) -> ()  [unwired: 2 in, 2 out]
            n129 = property on="Test Ring" class="Ring (strict)"("Visible"=w238) -> ()  [unwired: 2 in, 2 out]
          }
          frame "Relay", "Solenoid" {
            w241 = FALSE ("Visible")
            n130 = property on="Motor" class="Clust (strict)"("Visible"=w241) -> ()  [unwired: 2 in, 2 out]
            n131 = property on="Test Slider" class="Slide (strict)"("Visible"=w241) -> ()  [unwired: 2 in, 2 out]
            n132 = Search and Replace String(input string=w242, search string="/Value  **", replace string="/Direction") -> (result string=w248:string)  [unwired: 5 in, 3 out]
            n133 = property on="Test Ring" class="Ring (strict)"("Visible"=w241) -> ()  [unwired: 2 in, 2 out]
            n134 = call <vilib>:"NT Read String.vi"("Name"=w248) -> ("String"=w246:string)  [unwired: 9 in, 1 out]
            n135 = Equal?(x="Both directions", y=w246) -> (x = y?=w244:bool)
            n136 = Not(x=w244) -> (.not. x?=w245:bool)
            n137 = property on="Rev/Fwd" class="Clust (strict)"("Visible"=w244) -> ()  [unwired: 2 in, 2 out]
            n138 = property on="On/Off" class="Bool (strict)"("Visible"=w245, "Caption.Text"=w243) -> ()  [unwired: 2 in, 2 out]
          }
          frame "Compressor", "Digital Out" {
            w251 = FALSE ("Visible")
            # "Get direction and finish"
            n139 = property on="Motor" class="Clust (strict)"("Visible"=w251) -> ()  [unwired: 2 in, 2 out]
            n140 = property on="Test Slider" class="Slide (strict)"("Visible"=w251) -> ()  [unwired: 2 in, 2 out]
            n141 = property on="Test Ring" class="Ring (strict)"("Visible"=w251) -> ()  [unwired: 2 in, 2 out]
            n142 = property on="On/Off" class="Bool (strict)"("Visible"=TRUE, "Caption.Text"=w252) -> ()  [unwired: 2 in, 2 out]
            n143 = property on="Rev/Fwd" class="Clust (strict)"("Visible"=FALSE) -> ()  [unwired: 2 in, 2 out]
          }
          frame "Camera" {
            n144 = call <vilib>:"Get Last Path Segment.vi"("String in"=w259) -> ("String out"=w260:string)  [unwired: 10 in]
            n145 = property on="On/Off" class="Bool (strict)"("Visible"=FALSE) -> ()  [unwired: 2 in, 2 out]
            n146 = property on="Motor" class="Clust (strict)"("Visible"=FALSE) -> ()  [unwired: 2 in, 2 out]
            n147 = property on="Rev/Fwd" class="Clust (strict)"("Visible"=FALSE) -> ()  [unwired: 2 in, 2 out]
            n148 = case shown="\"White Balance  **\"" w260 {
              tunnel: w259 -> [w266 w275 w284 w293 w302 _ w308]
              tunnel: w258 -> [w264 w272 w281 w290 w299 _ _]
              frame "Size  **" {
                n149 = Index Array(array=w264) -> (element=w263:cluster{string[]})  [unwired: 1 in]
                n150 = call <vilib>:"NT Read String.vi"("Name"=w266) -> ("String"=w265:string)  [unwired: 9 in, 1 out]
                n151 = Unbundle(w263) -> (w261:string[])
                n152 = Match First String(2:w261, 3:w265) -> (0:w262:i32)  [unwired: 1 out]
                n153 = property on="Test Ring" class="Ring (strict)"("Value"=w262, "Strings []"=w261) -> ()  [unwired: 2 in, 2 out]
                n154 = property on="Test Ring" class="Ring (strict)"("Visible"=TRUE) -> ()  [unwired: 2 in, 2 out]
                n155 = property on="Test Slider" class="Slide (strict)"("Visible"=FALSE) -> ()  [unwired: 2 in, 2 out]
              }
              frame "White Balance  **" {
                n156 = Index Array(array=w272, index=1) -> (element=w273:cluster{string[]})
                n157 = call <vilib>:"NT Read String.vi"("Name"=w275) -> ("String"=w274:string)  [unwired: 9 in, 1 out]
                n158 = Unbundle(w273) -> (w270:string[])
                n159 = Match First String(2:w270, 3:w274) -> (0:w269:i32)  [unwired: 1 out]
                n160 = property on="Test Ring" class="Ring (strict)"("Value"=w269, "Strings []"=w270) -> ()  [unwired: 2 in, 2 out]
                n161 = property on="Test Ring" class="Ring (strict)"("Visible"=TRUE) -> ()  [unwired: 2 in, 2 out]
                n162 = property on="Test Slider" class="Slide (strict)"("Visible"=FALSE) -> ()  [unwired: 2 in, 2 out]
              }
              frame "Exposure  **" {
                n163 = Index Array(array=w281, index=2) -> (element=w282:cluster{string[]})
                n164 = call <vilib>:"NT Read String.vi"("Name"=w284) -> ("String"=w283:string)  [unwired: 9 in, 1 out]
                n165 = Unbundle(w282) -> (w278:string[])
                n166 = Match First String(2:w278, 3:w283) -> (0:w279:i32)  [unwired: 1 out]
                n167 = property on="Test Ring" class="Ring (strict)"("Value"=w279, "Strings []"=w278) -> ()  [unwired: 2 in, 2 out]
                n168 = property on="Test Ring" class="Ring (strict)"("Visible"=TRUE) -> ()  [unwired: 2 in, 2 out]
                n169 = property on="Test Slider" class="Slide (strict)"("Visible"=FALSE) -> ()  [unwired: 2 in, 2 out]
              }
              frame "Exposure Priority  **" {
                n170 = Index Array(array=w290, index=3) -> (element=w291:cluster{string[]})
                n171 = call <vilib>:"NT Read String.vi"("Name"=w293) -> ("String"=w292:string)  [unwired: 9 in, 1 out]
                n172 = Unbundle(w291) -> (w287:string[])
                n173 = Match First String(2:w287, 3:w292) -> (0:w288:i32)  [unwired: 1 out]
                n174 = property on="Test Ring" class="Ring (strict)"("Value"=w288, "Strings []"=w287) -> ()  [unwired: 2 in, 2 out]
                n175 = property on="Test Ring" class="Ring (strict)"("Visible"=TRUE) -> ()  [unwired: 2 in, 2 out]
                n176 = property on="Test Slider" class="Slide (strict)"("Visible"=FALSE) -> ()  [unwired: 2 in, 2 out]
              }
              frame "Color Enable  **" {
                n177 = Index Array(array=w299, index=4) -> (element=w300:cluster{string[]})
                n178 = call <vilib>:"NT Read String.vi"("Name"=w302) -> ("String"=w301:string)  [unwired: 9 in, 1 out]
                n179 = Unbundle(w300) -> (w296:string[])
                n180 = Match First String(2:w296, 3:w301) -> (0:w297:i32)  [unwired: 1 out]
                n181 = property on="Test Ring" class="Ring (strict)"("Value"=w297, "Strings []"=w296) -> ()  [unwired: 2 in, 2 out]
                n182 = property on="Test Ring" class="Ring (strict)"("Visible"=TRUE) -> ()  [unwired: 2 in, 2 out]
                n183 = property on="Test Slider" class="Slide (strict)"("Visible"=FALSE) -> ()  [unwired: 2 in, 2 out]
              }
              frame Default {
                n184 = property on="Test Ring" class="Ring (strict)"("Visible"=FALSE) -> ()  [unwired: 2 in, 2 out]
                n185 = property on="Test Slider" class="Slide (strict)"("Visible"=FALSE) -> ()  [unwired: 2 in, 2 out]
              }
              frame "Brightness  **", "Color Level  **", "Compression  **", "FPS  **", "Sharpness  **" {
                n186 = call <vilib>:"NT Read Number.vi"("Name"=w308) -> ("Numeric"=w307:dbl)  [unwired: 9 in, 1 out]
                n187 = local write "Test Slider"(w307) -> ()
                n188 = property on="Test Slider" class="Slide (strict)"("Visible"=TRUE, "Scale.Maximum"=100.0 ("Scale.Range:Maximum")) -> ()  [unwired: 2 in, 2 out]
                n189 = property on="Test Ring" class="Ring (strict)"("Visible"=FALSE) -> ()  [unwired: 2 in, 2 out]
              }
            }
          }
        }
        n190 = property on="Progress" class="Clust (strict)"("Visible"=FALSE) -> ()  [unwired: 2 in, 2 out]
      }
      event "Test Name": Mouse Enter {
        # "Populate the ring with the list of tests"
        n191 = event-data() -> ()  [unwired: 1 in, 1 out]
        n192 = call <vilib>:"NT Read String Array.vi"("Name"="TestMode/TestList") -> ("String Array"=w316:string[])  [unwired: 9 in, 1 out]
        n193 = Build Array (concatenate)("Select the test to run...", w316) -> (w315:string[])
        n194 = property on="Test Name" class="Ring (strict)"("Strings []"=w315) -> ()  [unwired: 2 in, 2 out]
      }
      event "Test Name": Value Change {
        w318 = FALSE ("Visible")
        # "Tell the robot the test name to run"
        n195 = event-data() -> ("NewVal"=w322:u16)  [unwired: 1 in]
        n196 = property on="Test Name" class="Ring (strict)"() -> ("Strings []"=w323:string[])  [unwired: 2 in, 2 out]
        n197 = local write "Progress"(T10 {"Test Progress"=0, "Test Progress Text"=""} ("Progress")) -> ()
        n198 = Index Array(array=w323, index=w322) -> (element=w321:string)
        n199 = call <vilib>:"NT Write String.vi"("String"=w321, "Name"="TestMode/TestName") -> ()  [unwired: 9 in, 1 out]
        n200 = property on="Progress" class="Clust (strict)"("Visible"=TRUE) -> ()  [unwired: 2 in, 2 out]
        n201 = property on="Motor" class="Clust (strict)"("Visible"=w318) -> ()  [unwired: 2 in, 2 out]
        n202 = property on="Test Slider" class="Slide (strict)"("Visible"=w318) -> ()  [unwired: 2 in, 2 out]
        n203 = property on="On/Off" class="Bool (strict)"("Visible"=w318) -> ()  [unwired: 2 in, 2 out]
        n204 = property on="Rev/Fwd" class="Clust (strict)"("Visible"=w318) -> ()  [unwired: 2 in, 2 out]
        n205 = property on="Test Ring" class="Ring (strict)"("Visible"=w318) -> ()  [unwired: 2 in, 2 out]
      }
      event "Listbox": Double Click {
        n206 = event-data() -> ("PlatMods.Shift"=w326:bool, "Row"=w328:i32)  [unwired: 1 in]
        n207 = case shown="True" w326 {
          tunnel: w328 -> [w332 _]
          tunnel: 1 -> [w331 _]
          frame False {
            n208 = property on="Listbox" class="LstBox (strict)"() -> ("Item Symbols"=w330:i32[])  [unwired: 2 in, 2 out]
            n209 = Replace Array Subset(array=w330, new element=w331, index=w332) -> (w329:i32[])
            n210 = property on="Listbox" class="LstBox (strict)"("Item Symbols"=w329) -> ()  [unwired: 2 in, 2 out]
          }
          frame True {
            w333 = 0 ("Top Row")
            n211 = property on="Listbox" class="LstBox (strict)"() -> ("Number of Rows"=w335:u32)  [unwired: 2 in, 2 out]
            n212 = Initialize Array(0, w335) -> (w334:i32[])
            n213 = property on="Listbox" class="LstBox (strict)"("Top Row"=w333, "Value"=w333, "Item Symbols"=w334) -> ()  [unwired: 2 in, 2 out]
          }
        }
      }
      event "Listbox": Key Down {
        n214 = event-data() -> ("VKey"=w339:T22)  [unwired: 1 in]
        n215 = case shown="\"Left\", \"Right\"" w339 {
          selector: w339 -> [w344 _]
          tunnel: eventvkey."Left" ("VKey") -> [w342 _]
          frame "Left", "Right" {
            n216 = Equal?(x=w342, y=w344) -> (x = y?=w343:bool)
            n217 = Select(t=0, s=w343, f=1) -> (s? t:f=w345:i32)
            n218 = property on="Listbox" class="LstBox (strict)"() -> ("Item Symbols"=w348:i32[])  [unwired: 2 in, 2 out]
            n219 = Replace Array Subset(array=w348, new element=w345, index="Listbox") -> (w347:i32[])
            n220 = property on="Listbox" class="LstBox (strict)"("Item Symbols"=w347) -> ()  [unwired: 2 in, 2 out]
          }
          frame Default {
          }
        }
      }
      event "DB Camera Config": Value Change {
        n221 = event-data() -> ("NewVal"=w352:bool)  [unwired: 1 in]
        n222 = case shown="False" w352 {
          tunnel: w351 -> [w361 _]
          tunnel: [w354 w372] -> w350
          tunnel: w349 -> [w353 w372]
          frame False {
            w368 = "Camera"
            w371 = FALSE ("Visible")
            n223 = local read "Camera Settings"() -> (w360:T2)
            n224 = Index Array(array=w361) -> (element=w364:cluster{string[]})  [unwired: 1 in]
            n225 = Unbundle(w360) -> ("Frame Rate"=w359:i32, "Compression"=w358:i32, "Size"=w362:u16)
            n226 = Unbundle(w364) -> (w363:string[])
            n227 = Index Array(array=w363, index=w362) -> (element=w357:string)
            n228 = call-poly <vilib>:"Write Key.vi"("section"=w368, "value"=w357, "key"="Size", "refnum"=w353) -> ("refnum out"=w370:T21)  [unwired: 2 in, 5 out]
            n229 = call-poly <vilib>:"Write Key.vi"("section"=w368, "value"=w359, "key"="FrameRate", "refnum"=w370) -> ("refnum out"=w369:T21)  [unwired: 1 in, 6 out]
            n230 = property on="Camera Settings" class="Clust (strict)"("Visible"=w371) -> ()  [unwired: 2 in, 2 out]
            n231 = local write "DB Camera Config"(w371) -> ()
            n232 = call-poly <vilib>:"Write Key.vi"("section"=w368, "value"=w358, "key"="Compression", "refnum"=w369) -> ("refnum out"=w355:T21)  [unwired: 1 in, 6 out]
            n233 = call <vilib>:"Close Config Data.vi"("refnum"=w355) -> ("file path"=w356:path)  [unwired: 2 in, 8 out]
            n234 = call <vilib>:"Open Config Data.vi"("configuration file path"=w356) -> ("refnum"=w354:T21)  [unwired: 8 in, 2 out]
          }
          frame True {
            n235 = property on="Camera Settings" class="Clust (strict)"("Visible"=TRUE) -> ()  [unwired: 2 in, 2 out]
          }
        }
      }
      event "Camera Settings": Value Change {
        n236 = event-data() -> ("NewVal"=w385:T2)  [unwired: 1 in]
        n237 = Index Array(array=w381) -> (element=w380:cluster{string[]})  [unwired: 1 in]
        n238 = Unbundle(w385) -> ("Frame Rate"=w376:i32, "Compression"=w375:i32, "Size"=w378:u16)
        n239 = Unbundle(w380) -> (w379:string[])
        n240 = Index Array(array=w379, index=w378) -> (element=w377:string)
        n241 = Format Into String(format string="%s   %dfps   %d%%", w377, w376, w375) -> (resulting string=w382:string)  [unwired: 2 in, 1 out]
        n242 = Build Array(w382) -> (w383:string[])
        n243 = property on="DB Camera Config" class="Bool (strict)"("Strings [4]"=w383) -> ()  [unwired: 2 in, 2 out]
      }
      event "Motor.Enable": Value Change {
        n244 = event-data() -> ("NewVal"=w391:bool)  [unwired: 1 in]
        n245 = Unbundle("Motor") -> ("Value"=w390:dbl)  [unwired: 1 out]
        n246 = Select(t=w390, s=w391, f=0.0) -> (s? t:f=w388:dbl)
        n247 = call <vilib>:"NT Write Number.vi"("Numeric"=w388, "Name"=w387) -> ()  [unwired: 9 in, 1 out]
      }
      event "Test Slider": Value Change {
        n248 = event-data() -> ("NewVal"=w394:dbl)  [unwired: 1 in]
        n249 = call <vilib>:"NT Write Number.vi"("Numeric"=w394, "Name"=w395) -> ()  [unwired: 9 in, 1 out]
      }
      event "On/Off": Value Change {
        n250 = event-data() -> ("NewVal"=w399:bool)  [unwired: 1 in]
        n251 = Boolean To (0,1)(Boolean=w399) -> (0, 1=w398:i16)
        n252 = call <vilib>:"NT Write Number.vi"("Numeric"=w398, "Name"=w397) -> ()  [unwired: 9 in, 1 out]
      }
      event "Rev/Fwd": Value Change {
        n253 = event-data() -> ("NewVal.Forward"=w407:bool, "NewVal.Reverse"=w406:bool)  [unwired: 1 in]
        n254 = Boolean To (0,1)(Boolean=w407) -> (0, 1=w403:i16)
        n255 = Boolean To (0,1)(Boolean=w406) -> (0, 1=w405:i16)
        n256 = Negate(x=w405) -> (-x=w404:i16)
        n257 = Add(x=w403, y=w404) -> (x+y=w402:i16)
        n258 = call <vilib>:"NT Write Number.vi"("Numeric"=w402, "Name"=w401) -> ()  [unwired: 9 in, 1 out]
      }
      event "Test Ring": Value Change {
        n259 = event-data() -> ("NewVal"=w411:u16)  [unwired: 1 in]
        n260 = property on="Test Ring" class="Ring (strict)"() -> ("Strings []"=w412:string[])  [unwired: 2 in, 2 out]
        n261 = Index Array(array=w412, index=w411) -> (element=w410:string)
        n262 = call <vilib>:"NT Write String.vi"("String"=w410, "Name"=w409) -> ()  [unwired: 9 in, 1 out]
      }
      event "Rec Mode": Value Change {
        # "Update globals for recording mode and path to read log from.\nClear when logging and let NetworkTables set path for vision to\nuse."
        n263 = event-data() -> ("NewVal"=w422:enum32{"Stop", "Record", "Playback"})  [unwired: 1 in]
        n264 = global write "WPI_DashboardLogging Global.vi" "Logging Filename"(path "") -> ()
        n265 = case shown="\"Stop\", \"Record\"" w422 {
          tunnel: w421 -> [_ w424 w432]
          tunnel: [_ _ w431] -> w418
          tunnel: [_ _ w430] -> _
          tunnel: w416 -> [_ _ w428]
          tunnel: cluster{i32, i32} {-250, 170} -> [_ _ w427]
          tunnel: [_ _ T23 {"Image Size"=TRUE, "Image Type"=TRUE, "Pixel Value"=TRUE, "ROI Information"=TRUE, "Zoom Factor"=FALSE} ("Image Information Shown:All Elements")] -> w414
          tunnel: [_ _ TRUE ("Zoom Factor")] -> w413
          frame Default {
          }
          frame "Stop", "Record" {
            # "Place Window too"
            n266 = invoke class="VI" method="FP.Close"(reference=w424) -> (reference out=w423:refnum<vi>)  [unwired: 2 in, 2 out]
            n267 = invoke class="VI" method="Abort VI"(reference=w423) -> ()  [unwired: 2 in, 3 out]
          }
          frame "Playback" {
            n268 = call "Open Playback Panel.vi"("Offset"=w427, "DB VI Ref"=w428, "Playback in"=w432) -> ("Playback out"=w429:refnum<vi>)  [unwired: 8 in]
            n269 = register-events(w429) -> (reference out=w431:refnum<event-registration>, error out=w430:errorcluster)  [unwired: 2 in]
          }
        }
        n270 = global write "WPI_DashboardLogging Global.vi" "Recording"(w422) -> ()
        n271 = property on="Camera Image" class="ImageControl"("Image Information Shown"=w414, "Image Information Visible"=w413) -> ()  [unwired: 2 in, 2 out]
        n272 = call <vilib>:"WPI_DashboardNT Log FieldName Cache.vi"("Operation"=enum16{"Lookup/Add", "Index", "Clear"}."Clear") -> ()  [unwired: 8 in, 3 out]
      }
      event Panel Close {
        w433 = enum32{"Stop", "Record", "Playback"}."Stop" ("Rec Mode")
        n273 = event-data() -> ()  [unwired: 1 in, 4 out]
        n274 = local write "Rec Mode"(w433) -> ()
        n275 = global write "WPI_DashboardLogging Global.vi" "Recording"(w433) -> ()
      }
      event Panel Close {
        # "Abort playback window and ourself"
        n276 = event-data() -> ()  [unwired: 1 in, 4 out]
        n277 = invoke class="VI" method="FP.Close"(reference=w438) -> (reference out=w437:refnum<vi>)  [unwired: 2 in, 2 out]
        n278 = invoke class="VI" method="Abort VI"(reference=w437) -> (error out=w436:errorcluster)  [unwired: 2 in, 2 out]
        n279 = invoke class="VI" method="Abort VI"(error in=w436) -> ()  [unwired: 2 in, 3 out]
      }
    }
  }
  n280 = property on="On/Off" class="Bool (strict)"("Visible"=w25) -> ()  [unwired: 2 in, 2 out]
  n281 = property on="Motor" class="Clust (strict)"("Visible"=w25) -> ()  [unwired: 2 in, 2 out]
  n282 = property on="Progress" class="Clust (strict)"("Visible"=w25) -> ()  [unwired: 2 in, 2 out]
  n283 = property on="Test Ring" class="Ring (strict)"("Visible"=w25) -> ()  [unwired: 2 in, 2 out]
  n284 = property on="Rev/Fwd" class="Clust (strict)"("Visible"=w25) -> ()  [unwired: 2 in, 2 out]
  n285 = property on="Camera Settings" class="Clust (strict)"("Visible"=w25) -> ()  [unwired: 2 in, 2 out]
  n286 = local write "DB Camera Config"(w25) -> ()
  n287 = global write "WPI_DashboardLogging Global.vi" "Recording"(w8) -> ()
  n288 = local write "Rec Mode"(w8) -> ()
